vi "DRT_Query.vi"(0 "System no.":i32=1 min=1 max=4 step=1, 2 "Rec. table to query":i32[](array[numeric]), 3 "With Rec. table IDs?":bool, 5 "error in":errorcluster) -> (14 "Trigger source":i32[](array[numeric]), 15 "Value":string[](array[string]), 19 "error out":errorcluster)   [LabVIEW 2020]
doc: "Returns the Data Recorder Trigger source and value for the queried data recorder tables.\n\nE-712, E-725, E-753: \n\nC-887, F-206, M-8X0: Only for GCS syntax version = GCS 2.0 or higher (check with CSV?.vi. If CSV?.vi is not supported, syntax version is GCS 1.0)."
panel:
  # "Returns the Data Recorder Trigger source and value for the queried data recorder tables."
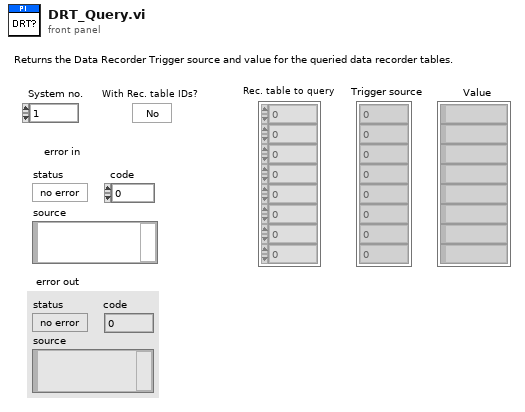
[diagram p1: front panel]
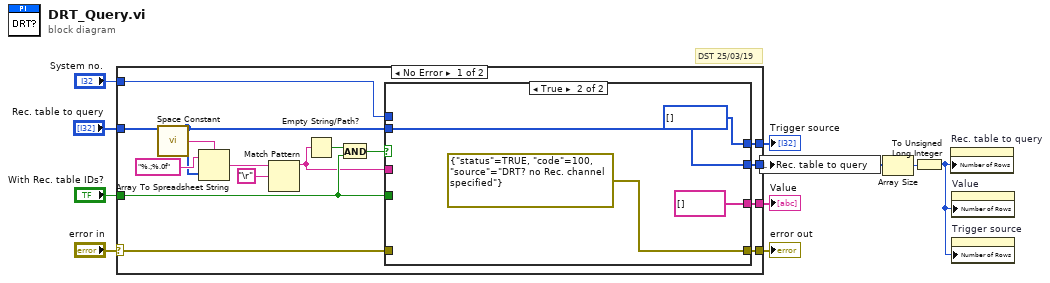
[diagram p0: block diagram]
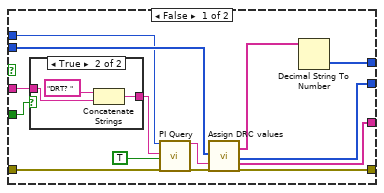
[diagram p2: hidden frame]
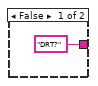
[diagram p3: hidden frame]
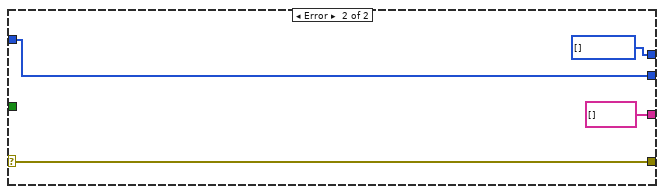
[diagram p4: hidden frame]
diagram:
  # "DST 25/03/19"
  n1 = case shown="No Error" "error in" {
    selector: "error in" -> [w12 w49]
    tunnel: "Rec. table to query" -> [w17 w48]
    tunnel: "System no." -> [w23 _]
    tunnel: [w25 w49] -> w8
    tunnel: [w24 i32[] [] ("Parameter values")] -> w7
    tunnel: [w18 string[] [] ("Source ID")] -> w6
    tunnel: "With Rec. table IDs?" -> [w15 _]
    tunnel: [w11 w48] -> w3
    frame No Error {
      n2 = call "Space Constant.vi"() -> ("String"=w21:string)
      n3 = Array To Spreadsheet String(delimiter (Tab)=w21, array=w17, 3:"%.;%.0f" ("Format String")) -> (spreadsheet string=w19:string)
      n4 = Match Pattern(string=w19, regular expression="\r") -> (before substring=w14:string)  [unwired: 4 out]
      n5 = Empty String/Path?(string/path=w14) -> (empty?=w13:bool)
      n6 = And(x=w13, y=w15) -> (x .and. y?=w16:bool)
      n7 = case shown="True" w16 {
        tunnel: w12 -> [w36 _]
        tunnel: w14 -> [w37 _]
        tunnel: w23 -> [w33 _]
        tunnel: [w35 errorcluster {"status"=TRUE, "code"=100, "source"="DRT? no Rec. channel specified"} ("error out")] -> w25
        tunnel: [w29 i32[] [] ("Parameter values")] -> w24
        tunnel: [w31 string[] [] ("Source ID")] -> w18
        tunnel: w17 -> [w34 w44]
        tunnel: w15 -> [w32 _]
        tunnel: [w26 w44] -> w11
        frame False {
          n8 = case shown="True" w32 {
            tunnel: ["DRT?" w42] -> w38
            tunnel: w37 -> [_ w41]
            frame False {
            }
            frame True {
              n9 = Concatenate Strings("DRT? ", w41) -> (w42:string)
            }
          }
          n10 = call "PI Query.vi"("System no."=w33, "String to send"=w38, "Attach termination char.?"=TRUE ("Attach Linefeed?"), "error in"=w36) -> ("String read"=w28:string, "error out"=w27:errorcluster)  [unwired: 3 in, 11 out]
          n11 = call "Assign DRC values.vi"("Queried Rec. table"=w34, "Input String"=w28, "error in"=w27) -> ("Source ID"=w30:string[], "Queried Rec. table out"=w26:i32[], "Rec. option string"=w31:string[], "error out"=w35:errorcluster)  [unwired: 1 in, 12 out]
          n12 = Decimal String To Number(string=w30) -> (number=w29:i32[])  [unwired: 3 out]
        }
        frame True {
        }
      }
    }
    frame Error {
    }
  }
  "Value" <- w6
  "error out" <- w8
  "Trigger source" <- w7
  n13 = local write "Rec. table to query"(w3) -> ()
  n14 = Array Size(array=w3) -> (size(s)=w2:i32)
  n15 = To Unsigned Long Integer(number=w2) -> (unsigned 32bit integer=w1:u32)
  n16 = property on="Rec. table to query" class="Arr (strict)"("Number of Rows"=w1) -> ()  [unwired: 2 in, 2 out]
  n17 = property on="Value" class="Arr (strict)"("Number of Rows"=w1) -> ()  [unwired: 2 in, 2 out]
  n18 = property on="Trigger source" class="Arr (strict)"("Number of Rows"=w1) -> ()  [unwired: 2 in, 2 out]
